vi "From JSON String.vi"(0 "Display State In":T1, 7 "JSON String":string, 9 "Container State":T2, 11 "error in (no error)":errorcluster) -> (4 "Display State Out":T1, 15 "error out":errorcluster)   [LabVIEW 2017, in "Variant Tree API.lvlib" / "Variant Tree.xctl"]
uses:
  Variant Tree.xctl
  <vilib>/_xctls/Container State.ctl
  State.ctl
  <vilib>/National Instruments/Variant JSON API/Variant JSON API.lvlib
  <vilib>/_xctls/XControlSupport.lvlib
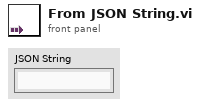
[diagram p1: front panel]
types:
  T1 = typedef "Variant Tree API.lvlib/Variant Tree.xctl/State.ctl" = cluster{"Numeric":dbl}
  T2 = typedef "XControlSupport.lvlib/Container State.ctl" = cluster{"Indicator?":bool, "Run Mode?":bool, " Refnum":refnum<vi>}
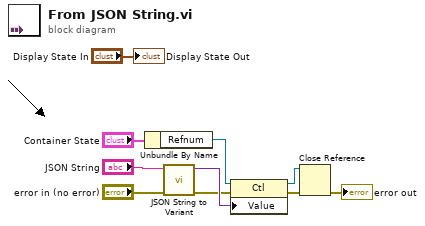
[diagram p0: block diagram]
diagram:
  n1 = Unbundle By Name("Container State") -> ("Refnum"=w8:refnum<vi>)
  n2 = call <vilib>:"JSON String to Variant.vi"("error in (no error)"="error in (no error)", "JSON String"="JSON String") -> ("error out"=w4:errorcluster, "Variant out"=w7:variant)  [unwired: 8 in]
  n3 = property class="Ctl"(reference=w8, error in=w4, "Value"=w7) -> (reference out=w1:refnum<vi>, error out=w3:errorcluster)
  n4 = Close Reference(reference=w1, error in (no error)=w3) -> (error out=→"error out":errorcluster)
  "Display State Out" <- "Display State In"
